vi "Run Test.vi"(8 "error in (no error)":errorcluster, 11 "Example Test In":refnum<class "Example Parallel Test.lvclass">) -> (0 "error out":errorcluster, 1 "Fail Codes":string[](array[string]), 2 "Tests Passed":bool[](array[boolean]), 3 "Example Test Out":refnum<class "Example Parallel Test.lvclass">)   [LabVIEW 2015]
uses:
  Test Class/Test Class.lvclass
  Classes/Application/Class/Application.lvclass
  Example Parallel Test.lvclass
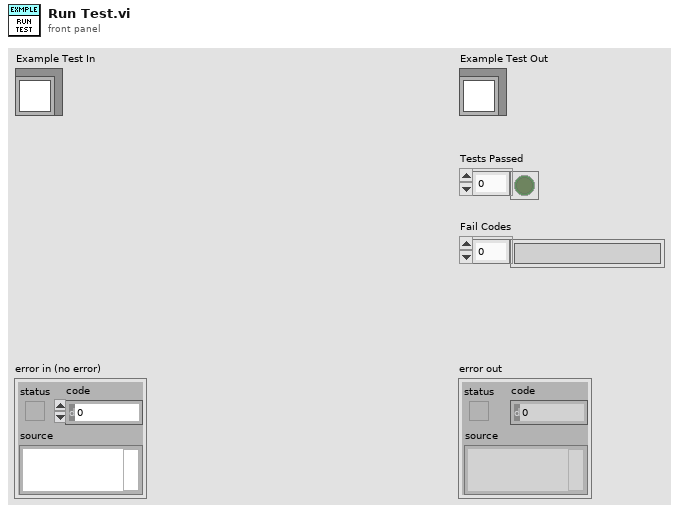
[diagram p1: front panel]
types:
  T1 = cluster{"Serial Number Reference":refnum<vi>, "Status Message Reference":refnum<vi>, "Position":u32}[]
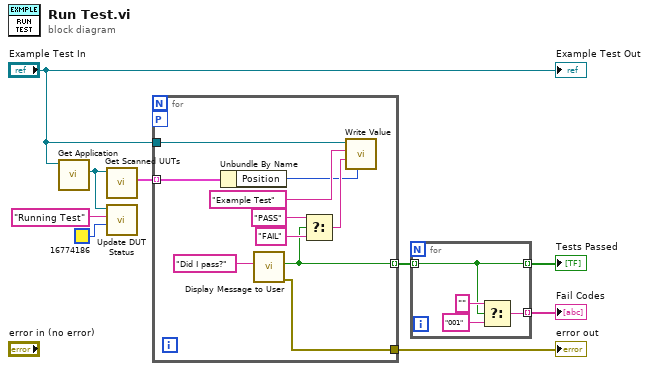
[diagram p0: block diagram]
diagram:
  n1 = call "Get Application.vi"("Test Class in"="Example Test In") -> ("Application.lvlib:Application.lvclass"=w2:refnum<class "Application.lvclass">)  [unwired: 9 in, 1 out]
  n2 = call-dynamic "Get Scanned UUTs.vi"("Application in"=w2) -> ("Active UUTs"=w3:T1)  [unwired: 8 in, 2 out]
  n3 = call "Update DUT Status.vi"("BG Color"=u32 16774186, "Message ('')"="Running Test", "Application in"=w2) -> ()  [unwired: 7 in, 2 out]
  n4 = for {
    tunnel: [w18] -> w9
    tunnel: [w15] -> w6 mode=indexing
    tunnel: w3 -> [w12] mode=indexing
    tunnel: "Example Test In" -> [w10]
    workers-P: _ -> [_]
    n5 = Unbundle By Name(w12) -> ("Position"=w11:u32)
    n6 = call "Display Message to User"("Message"="Did I pass?") -> ("error out"=w18:errorcluster, "OK"=w15:bool)  [unwired: 9 in]
    n7 = Select(t="PASS" ("Message"), s=w15, f="FAIL" ("Message")) -> (s? t:f=w13:string)
    n8 = call "Write Value.vi"("Position"=w11, "Value"=w13, "Label"="Example Test" ("Message"), "Test Class in"=w10) -> ()  [unwired: 7 in, 1 out]
  }
  "error out" <- w9
  n9 = for {
    tunnel: [w23] -> w5 mode=indexing
    tunnel: w6 -> [w20] mode=indexing
    tunnel: [w20] -> w4 mode=indexing
    n10 = Select(t="", s=w20, f="001") -> (s? t:f=w23:string)
  }
  "Tests Passed" <- w4
  "Fail Codes" <- w5
  "Example Test Out" <- "Example Test In"
